vi "all_VIs.vi"() -> ()   [LabVIEW 2014]
uses:
  SQLite3LV/SQLite3 Class/sqlite3.lvclass
  SQLite3LV/Cursor Class/cursor.lvclass
  SQLite3LV/Cursor Class/Fetch N - String.vi
  SQLite3LV/Cursor Class/Fetch N - DBL.vi
  SQLite3LV/Cursor Class/Fetch N - I32.vi
  SQLite3LV/Cursor Class/Fetch N - I64.vi
  SQLite3LV/Cursor Class/Fetch N - Blob.vi
panel:
  out "Array":T1(array[cluster])
  out "SQLite3LV:Cursor 3":refnum<class "cursor.lvclass">
  out "error out 2":errorcluster
  out "error out":errorcluster
  out "SQLite3LV:Cursor 3":refnum<class "cursor.lvclass">
  out "SQLite3LV:Cursor 3":refnum<class "cursor.lvclass">
  in  "SQLite3LV:Cursor 3":refnum<class "cursor.lvclass">
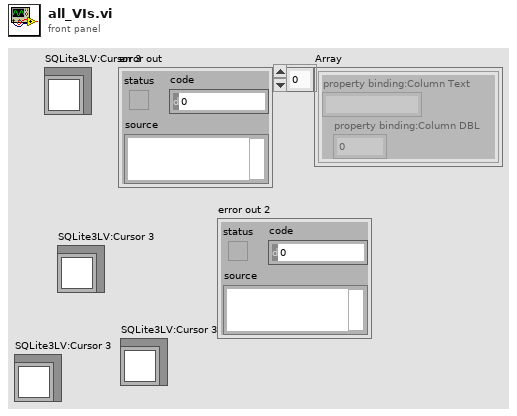
[diagram p1: front panel]
types:
  T1 = cluster{"property binding:Column Text":string, "property binding:Column DBL":dbl}[]
  T2 = cluster{"property binding:Column Text":string, "property binding:Column DBL":dbl}
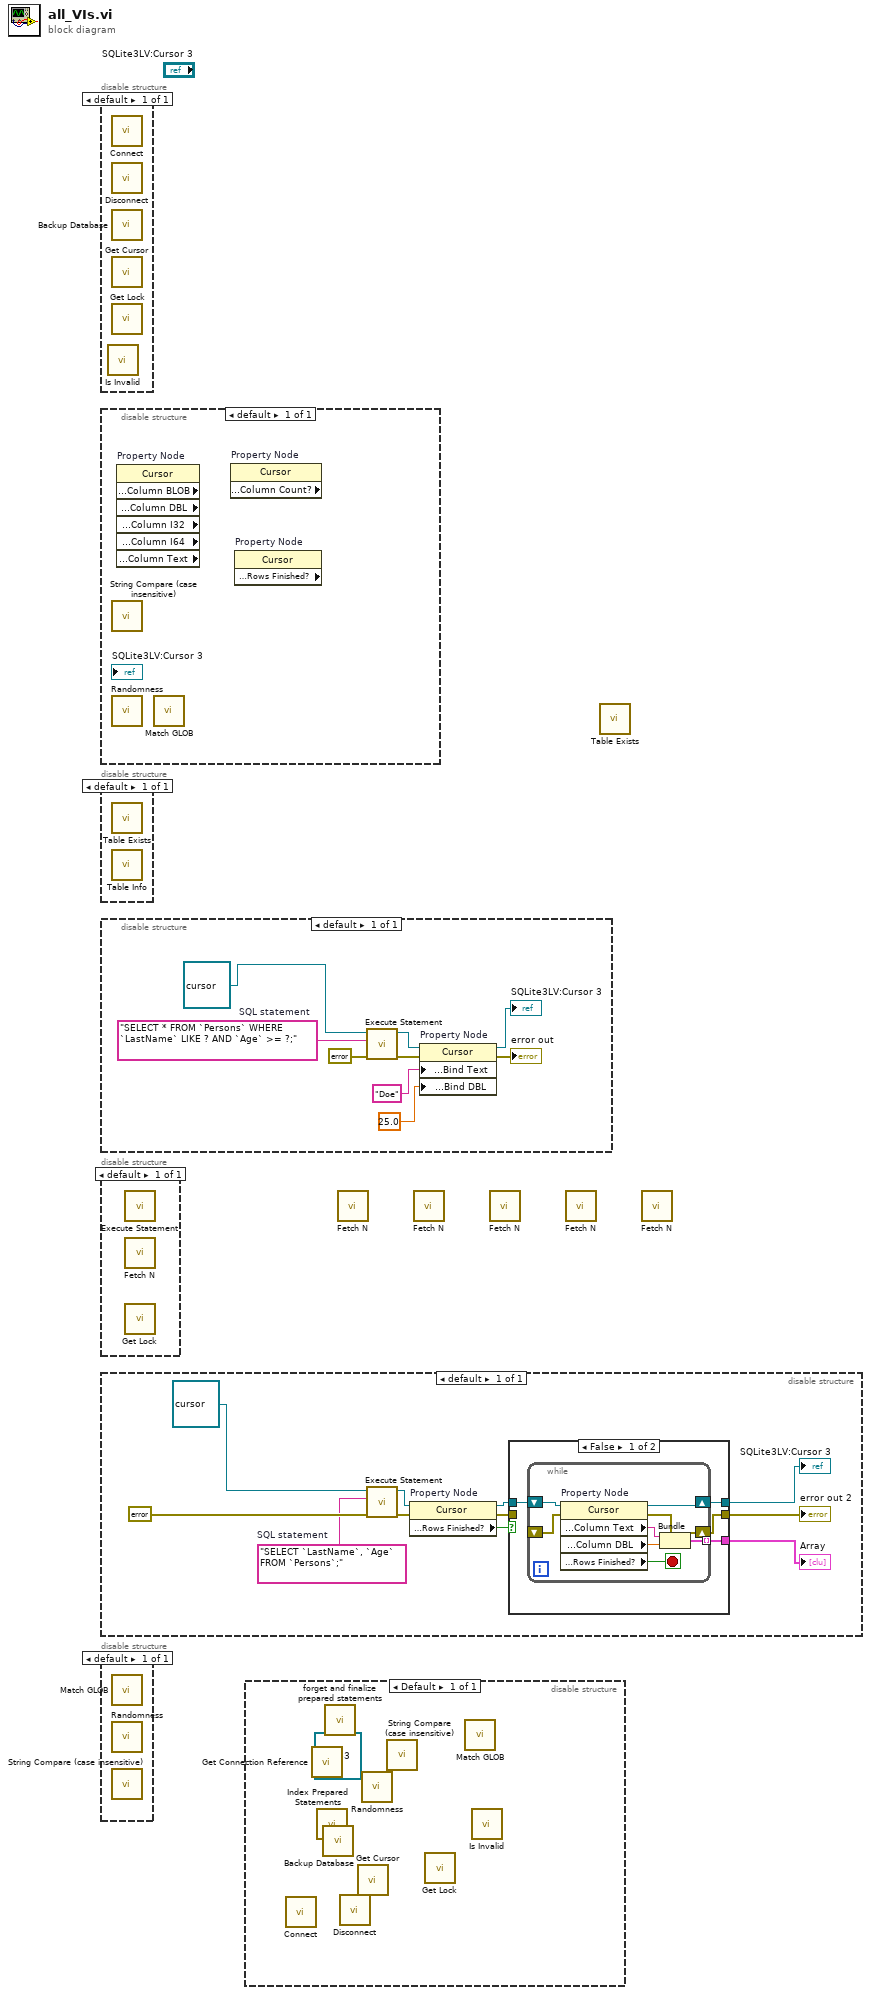
[diagram p0: block diagram]
diagram:
  n1 = disable-structure shown="default" {
    frame Enabled {
      n2 = call "Is Invalid.vi"() -> ()  [unwired: 4 in, 2 out]
      n3 = call "Connect.vi"() -> ()  [unwired: 10 in, 2 out]
      n4 = call "Disconnect.vi"() -> ()  [unwired: 11 in, 1 out]
      n5 = call "Backup Database.vi"() -> ()  [unwired: 9 in, 3 out]
      n6 = call "Get Cursor.vi"() -> ()  [unwired: 9 in, 3 out]
      n7 = call "Get Lock.vi"() -> ()  [unwired: 9 in, 3 out]
    }
  }
  n8 = disable-structure shown="default" {
    frame Enabled {
      n9 = call "String Compare (case insensitive).vi"() -> ()  [unwired: 10 in, 2 out]
      n10 = call "Randomness.vi"() -> ()  [unwired: 10 in, 2 out]
      n11 = property on="Property Node" class="Cursor" props=["property binding:Column BLOB", "property binding:Column DBL", "property binding:Column I32", "property binding:Column I64", "property binding:Column Text"]() -> ()  [unwired: 2 in, 7 out]
      n12 = call "Match GLOB.vi"() -> ()  [unwired: 10 in, 2 out]
      n13 = property on="Property Node" class="Cursor" props=["property binding:Column Count?"]() -> ()  [unwired: 2 in, 3 out]
      n14 = property on="Property Node" class="Cursor" props=["property binding:Rows Finished?"]() -> ()  [unwired: 2 in, 3 out]
    }
  }
  n15 = disable-structure shown="default" {
    frame Enabled {
      n16 = call "Table Exists.vi"() -> ()  [unwired: 9 in, 3 out]
      n17 = call "Table Info.vi"() -> ()  [unwired: 9 in, 3 out]
    }
  }
  n18 = disable-structure shown="default" {
    frame Enabled {
      w9 = "SELECT * FROM `Persons` WHERE `LastName` LIKE ? AND `Age` >= ?;"  # SQL statement
      n19 = call "Execute Statement.vi"("error in (no error)"=errorcluster {"status"=FALSE, "code"=0, "source"=""} ("error in"), "SQL statement"=w9, "SQLite3LV Cursor in"=refnum<class "cursor.lvclass"> refnum ("SQLite3LV:Cursor")) -> ("error out"=w7:errorcluster, "SQLite3LV Cursor out"=w8:refnum<class "cursor.lvclass">)  [unwired: 7 in]
      n20 = property on="Property Node" class="Cursor"(reference=w8, error in=w7, "property binding:Bind Text"="Doe" ("Bind Text"), "property binding:Bind DBL"=25.0 ("Bind DBL")) -> (reference out=→"SQLite3LV:Cursor 3":refnum<class "cursor.lvclass">, error out=→"error out":errorcluster)
    }
  }
  n21 = disable-structure shown="default" {
    frame Enabled {
      n22 = call "Execute Statement.vi"() -> ()  [unwired: 10 in, 2 out]
      n23 = call-poly "Fetch N.vi"() -> ()  [unwired: 8 in, 4 out]
      n24 = call "Get Lock.vi"() -> ()  [unwired: 9 in, 3 out]
    }
  }
  n25 = disable-structure shown="default" {
    frame Enabled {
      w17 = "SELECT `LastName`, `Age` FROM `Persons`;"  # SQL statement
      n26 = call "Execute Statement.vi"("error in (no error)"=errorcluster {"status"=FALSE, "code"=0, "source"=""} ("error in"), "SQL statement"=w17, "SQLite3LV Cursor in"=refnum<class "cursor.lvclass"> refnum ("SQLite3LV:Cursor 3")) -> ("error out"=w15:errorcluster, "SQLite3LV Cursor out"=w16:refnum<class "cursor.lvclass">)  [unwired: 7 in]
      n27 = property on="Property Node" class="Cursor"(reference=w16, error in=w15) -> (reference out=w13:refnum<class "cursor.lvclass">, error out=w14:errorcluster, "property binding:Rows Finished?"=w12:bool)
      n28 = case shown="False" w12 {
        tunnel: [w24 w33] -> w19
        tunnel: [w23 w34] -> w18
        tunnel: w14 -> [_ w33]
        tunnel: w13 -> [w22 w34]
        tunnel: [w21 _] -> w11
        frame False {
          n29 = while {
            tunnel: [w25] -> w21 mode=indexing
            shift-right: [w31] -> w23
            shift-left: w22 -> [w29]
            shift-right: [w32] -> w24
            shift-left: _ -> [w30]
            stop <- w28 stop-if-true
            n30 = property on="Property Node" class="Cursor"(reference=w29, error in=w30) -> (reference out=w31:refnum<class "cursor.lvclass">, error out=w32:errorcluster, "property binding:Column Text"=w27:string, "property binding:Column DBL"=w26:dbl, "property binding:Rows Finished?"=w28:bool)
            n31 = Bundle("property binding:Column Text"=w27, "property binding:Column DBL"=w26) -> (w25:T2)  [unwired: 1 in]
          }
        }
        frame True {
        }
      }
      "SQLite3LV:Cursor 3" <- w18
      "error out 2" <- w19
      "Array" <- w11
    }
  }
  n32 = disable-structure shown="default" {
    frame Enabled {
      n33 = call "Match GLOB.vi"() -> ()  [unwired: 10 in, 2 out]
      n34 = call "Randomness.vi"() -> ()  [unwired: 10 in, 2 out]
      n35 = call "String Compare (case insensitive).vi"() -> ()  [unwired: 10 in, 2 out]
    }
  }
  n36 = disable-structure shown="Default" {
    frame Enabled {
      (unwired) refnum<class "sqlite3.lvclass"> refnum ("SQLite3LV:SQLite3LV Connection")
      n37 = call "Connect.vi"() -> ()  [unwired: 10 in, 2 out]
      n38 = call "Get Connection Reference.vi"() -> ()  [unwired: 9 in, 3 out]
      n39 = call "Index Prepared Statements.vi"() -> ()  [unwired: 8 in, 4 out]
      n40 = call "Backup Database.vi"() -> ()  [unwired: 9 in, 3 out]
      n41 = call "forget and finalize prepared statements.vi"() -> ()  [unwired: 10 in, 2 out]
      n42 = call "Disconnect.vi"() -> ()  [unwired: 11 in, 1 out]
      n43 = call "Get Cursor.vi"() -> ()  [unwired: 9 in, 3 out]
      n44 = call "Randomness.vi"() -> ()  [unwired: 10 in, 2 out]
      n45 = call "String Compare (case insensitive).vi"() -> ()  [unwired: 10 in, 2 out]
      n46 = call "Get Lock.vi"() -> ()  [unwired: 9 in, 3 out]
      n47 = call "Match GLOB.vi"() -> ()  [unwired: 10 in, 2 out]
      n48 = call "Is Invalid.vi"() -> ()  [unwired: 4 in, 2 out]
    }
  }
  n49 = call-poly "Fetch N.vi"() -> ()  [unwired: 8 in, 4 out]
  n50 = call-poly "Fetch N.vi"() -> ()  [unwired: 8 in, 4 out]
  n51 = call-poly "Fetch N.vi"() -> ()  [unwired: 8 in, 4 out]
  n52 = call-poly "Fetch N.vi"() -> ()  [unwired: 8 in, 4 out]
  n53 = call "Table Exists.vi"() -> ()  [unwired: 9 in, 3 out]
  n54 = call-poly "Fetch N.vi"() -> ()  [unwired: 8 in, 4 out]
